vi "nowall move.vi"(7 "dir":enum16{"R", "L"}(ring), 8 "error in (no error)":errorcluster, 9 "Speed":dbl, 10 "Distance":dbl, 11 "IR if?":dbl) -> (0 "error out":errorcluster)   [LabVIEW 2019]
uses:
  <vilib>/Platform/TimedLoop/XDataNode/timing_clust.ctl
  <vilib>/Platform/TimedLoop/XDataNode/nitl_modes.ctl
  <vilib>/Platform/TimedLoop/XDataNode/wakeup.ctl
  <vilib>/platform/TimedLoop/XDataNode/XDataNode.xnode
  <vilib>/Platform/TimedLoop/XDataNode/XDNodeRunTimeDep.lvlib
panel:
  out "x > y?":bool
  out "x*y":dbl[](array[numeric])
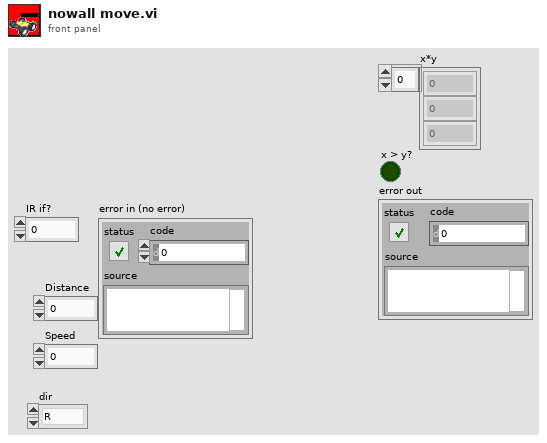
[diagram p1: front panel]
types:
  T1 = typedef "AI.lvlib/AI Reference.ctl" = cluster{"myRIO Reference":T2, "AI Channels List":T6, "AI Scaling Constants List":T8}
  T2 = typedef "myRIO Generic Hardware Reference.ctl" = cluster{"myRIO Model":T3, "myRIO Hardware Reference":T4}
  T3 = typedef "Hardware Version Enum.ctl" = enum16{"Unknown", "myRIO-1900", "myRIO-1950", "roboRIO", "NI ELVIS RIO CM", "ELVIS III"}
  T4 = typedef "myRIO v1.0 Reference.ctl" = cluster{"Generic FPGA Reference":T5, "Allow multiple opens":bool}
  T5 = typedef "Generic FPGA Reference.ctl" = refnum<k20>
  T6 = typedef "AI Channels List.ctl" = T7[]
  T7 = typedef "AI Channels Enum.ctl" = enum16{"Not Connected", "AudioIn/Left", "AudioIn/Right", "C/AI0", "C/AI1", "A/AI0", "A/AI1", "A/AI2", "A/AI3", "A/AI4", "A/AI5", "A/AI6", "A/AI7", "B/AI0", "B/AI1", "B/AI2", "B/AI3", "B/AI4", "B/AI5", "B/AI6", "B/AI7", "AI/AI0", "AI/AI1", "AI/AI2", "AI/AI3", "A/AI0 (DIFF)", "A/AI1 (DIFF)", "A/AI2 (DIFF)", "A/AI3 (DIFF)", "B/AI0 (DIFF)", "B/AI1 (DIFF)", "B/AI2 (DIFF)", "B/AI3 (DIFF)"}
  T8 = typedef "Analog Scaling Constants List.ctl" = T9[]
  T9 = typedef "Analog Scaling Constants.ctl" = cluster{"LSB Weight (Volts)":dbl, "Offset (Volts)":dbl, "Signed?":bool}
  T10 = typedef "XDNodeRunTimeDep.lvlib/timing_clust.ctl" = cluster{"Expected End [f-1]":u64, "Actual End [f-1]":u64, "Finished Late? [f-1]":bool, "Expected End [i-1]":u64, "Actual End [i-1]":u64, "Finished Late? [i-1]":bool, "Expected Start [i]":u64, "Actual Start [i]":u64, "Expected Start [f]":u64, "Actual Start [f]":u64, "Source Name":string, "Structure Name":string, "Period":i64, "Deadline":i64, "Offset":i64, "Start":i64, "Priority":i32, "Timeout":i32, "Mode":T11, "Wakeup Reason":T12, "Error":errorcluster, "Source Type":string, "Secondary Source Type":string, "Global End Time":u64, "Global Start Time":u64, "Frame Duration":u64, "Iteration Duration":u64, "Assigned CPU":i32, "I/O Scan Engine Mode":u32}
  T11 = typedef "XDNodeRunTimeDep.lvlib/nitl_modes.ctl" = enum32{"No Change", "Process missed periods, maintain original phase", "Discard missed periods, maintain original phase", "Process missed periods, ignore original phase", "Discard missed periods, ignore original phase"}
  T12 = typedef "XDNodeRunTimeDep.lvlib/wakeup.ctl" = enum32{"Normal", "Aborted", "Asynchronous wakeup", "Timing source error", "Timed loop error", "Timeout"}
  T13 = typedef "IR out.ctl" = cluster{"DC estimate (V) 2":dbl, "DC estimate (V)":dbl, "AC estimate (Vrms)":dbl, "AC estimate (Vrms) 2":dbl}
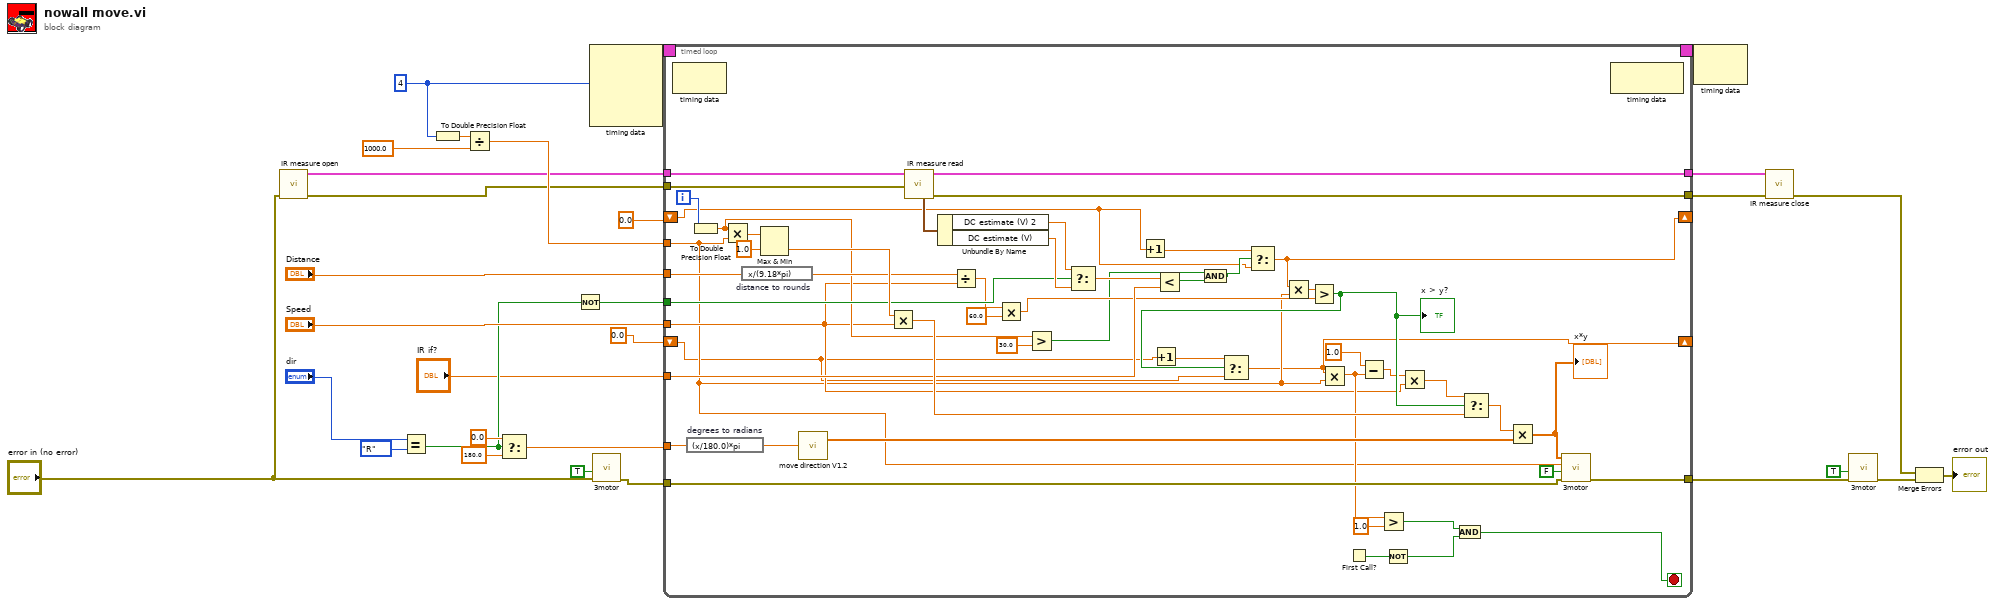
[diagram p0: block diagram]
diagram:
  w21 = i64 4 ("Period")
  n1 = call "IR measure open.vi"("error in (no error)"="error in (no error)") -> ("error out"=w16:errorcluster, "AI Ref Out"=w17:T1)  [unwired: 9 in]
  n2 = Equal?(x="dir", y=enum16{"R", "L"}."R") -> (x = y?=w15:bool)
  n3 = To Double Precision Float(number=w21) -> (double precision float=w20:dbl)
  n4 = Divide(x=w20, y=1000.0) -> (x/y=w18:dbl)
  n5 = Select(t=0.0, s=w15, f=180.0) -> (s? t:f=w26:dbl)
  n6 = Not(x=w15) -> (.not. x?=w6:bool)
  n7 = node-c288(w21) -> (w28:T10)  [unwired: 3 in]
  n8 = call "3motor.vi"("error in (no error)"="error in (no error)", "Reset"=TRUE) -> ("error out"=w13:errorcluster)  [unwired: 9 in]
  n9 = timed-loop {
    timing: w28 -> [_]
    timing-out: [_] -> w27
    tunnel: w26 -> [w59]
    tunnel: "Speed" -> [w41]
    tunnel: "Distance" -> [w75]
    tunnel: w18 -> [w39]
    tunnel: w17 -> [w74]
    tunnel: w16 -> [w73]
    tunnel: w6 -> [w69]
    tunnel: "IR if?" -> [w67]
    tunnel: w13 -> [w63]
    tunnel: [w62] -> w10
    tunnel: [w61] -> w9
    tunnel: [w60] -> w8
    shift-right: [w33] -> _
    shift-left: 0.0 -> [w34]
    shift-right: [w31] -> _
    shift-left: 0.0 -> [w32]
    i -> [w82]
    stop <- w35 stop-if-true
    n10 = node-c288() -> ()  [unwired: 1 in, 1 out]
    n11 = expression code="(x/180.0)*pi" "degrees to radians"(w59) -> (w58:dbl)
    n12 = To Double Precision Float(number=w82) -> (double precision float=w46:dbl)
    n13 = Multiply(x=w46, y=w39) -> (x*y=w81:dbl)
    n14 = expression code="x/(9.18*pi)" "distance to rounds"(w75) -> (w77:dbl)
    n15 = Max & Min(x=w81, y=1.0) -> (min(x,y)=w79:dbl)  [unwired: 1 out]
    n16 = call "move direction V1.2.vi"("theta"=w58) -> ("out array"=w78:dbl[])  [unwired: 1 out]
    n17 = Multiply(x=w79, y=w41) -> (x*y=w76:dbl)
    n18 = call "IR measure read.vi"("error in (no error)"=w73, "AI Ref In"=w74) -> ("error out"=w62:errorcluster, "AI Ref Out"=w61:T1, "output cluster"=w72:T13)  [unwired: 6 in, 1 out]
    n19 = Unbundle By Name(w72) -> ("DC estimate (V) 2"=w71:dbl, "DC estimate (V)"=w70:dbl)
    n20 = Divide(x=w77, y=w41) -> (x/y=w66:dbl)
    n21 = Multiply(x=w66, y=60.0) -> (x*y=w64:dbl)
    n22 = Greater?(x=w46, y=30.0) -> (0:w44:bool)
    n23 = Select(t=w71, s=w69, f=w70) -> (s? t:f=w68:dbl)
    n24 = Increment(x=w34) -> (x+1=w56:dbl)
    n25 = Increment(x=w32) -> (x+1=w55:dbl)
    n26 = Less?(x=w68, y=w67) -> (x < y?=w43:bool)
    n27 = And(x=w44, y=w43) -> (x .and. y?=w42:bool)
    n28 = Select(t=w56, s=w42, f=w34) -> (s? t:f=w33:dbl)
    n29 = Multiply(x=w33, y=w39) -> (x*y=w40:dbl)
    n30 = Greater?(x=w40, y=w64) -> (0:w53:bool)
    "x > y?" <- w53
    n31 = Select(t=w55, s=w53, f=w32) -> (s? t:f=w31:dbl)
    n32 = Multiply(x=w31, y=w39) -> (x*y=w50:dbl)
    n33 = First Call?() -> (First Call?: T/F=w38:bool)
    n34 = Subtract(x=1.0, y=w50) -> (x-y=w52:dbl)
    n35 = Greater?(x=w50, y=1.0) -> (0:w37:bool)
    n36 = Not(x=w38) -> (.not. x?=w36:bool)
    n37 = Multiply(x=w52, y=w41) -> (x*y=w51:dbl)
    n38 = And(x=w37, y=w36) -> (x .and. y?=w35:bool)
    n39 = Select(t=w51, s=w53, f=w76) -> (s? t:f=w57:dbl)
    n40 = Multiply(x=w57, y=w78) -> (x*y=w48:dbl[])
    "x*y" <- w48
    n41 = call "3motor.vi"("error in (no error)"=w63, "Reset"=FALSE, "dt(s)"=w39, "Motor speed"=w48) -> ("error out"=w60:errorcluster)  [unwired: 7 in]
    n42 = node-c288() -> ()  [unwired: 1 in, 1 out]
  }
  n43 = node-c288(w27) -> ()  [unwired: 1 out]
  n44 = call "IR measure close.vi"("error in (no error)"=w10, "AI Ref In"=w9) -> ("error out"=w4:errorcluster)  [unwired: 9 in]
  n45 = call "3motor.vi"("error in (no error)"=w8, "Reset"=TRUE) -> ("error out"=w5:errorcluster)  [unwired: 9 in]
  n46 = Merge Errors(w4, w5) -> (→"error out":errorcluster)
